vi "Close Device.vi"(8 "error in (no error)":errorcluster, 11 "Simulated Scope in":refnum<class "Simulated Scope.lvclass">) -> (0 "error out":errorcluster, 3 "Simulated Scope out":refnum<class "Simulated Scope.lvclass">)   [LabVIEW 2020, in "Simulated Scope.lvlib" / "Simulated Scope.lvclass"]
uses:
  Simulated Scope.lvclass
  Simulated Scope.lvclass/Simulated Scope.ctl
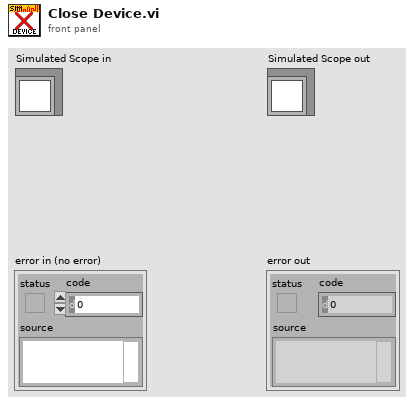
[diagram p1: front panel]
types:
  T1 = typedef "Simulated Scope.lvlib/Simulated Scope.lvclass/Ref Data.ctl" = cluster{"Sim Queue Name":string, "Waveform Queue":refnum<queue>}
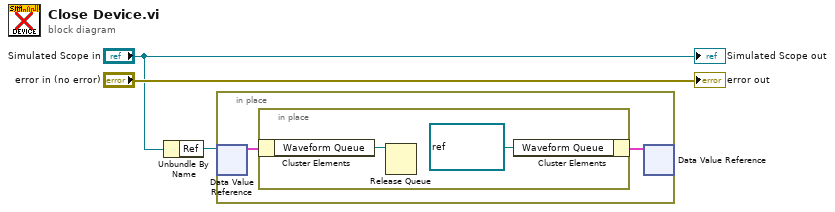
[diagram p0: block diagram]
diagram:
  n1 = Unbundle By Name("Simulated Scope in") -> ("Ref"=w2:refnum<data-value>)
  n2 = in-place {
    n3 = in-place-dvr #1(w2) -> (w5:T1)  [unwired: 1 out]
    n4 = in-place {
      n5 = in-place-cluster #2(w5) -> ("Waveform Queue"=w7:refnum<queue>)
      n6 = Release Queue(queue=w7) -> ()  [unwired: 2 in, 3 out]
      n7 = in-place-cluster #2("Waveform Queue"=refnum<queue> refnum) -> (w4:T1)
    }
    n8 = in-place-dvr #1(w4) -> ()  [unwired: 2 out]
  }
  "error out" <- "error in (no error)"
  "Simulated Scope out" <- "Simulated Scope in"
